vi "Dato_Booleano.vi"() -> ()   [LabVIEW 2016]
panel:
  in  "Boolean":bool
  in  "Stop Button":bool
  in  "STR1":string
  in  "DBL1":dbl
  in  "ARRAY1":dbl[](array[numeric])
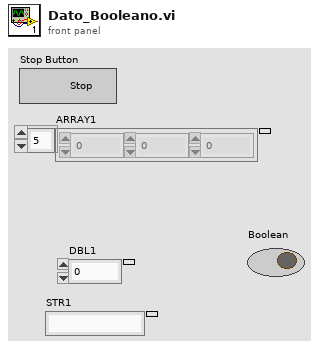
[diagram p1: front panel]
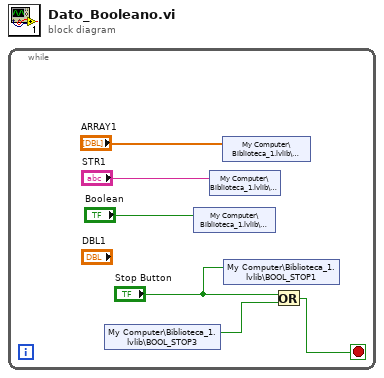
[diagram p0: block diagram]
diagram:
  n1 = while {
    stop <- w4 stop-if-true
    n2 = shared-variable "My Computer\\Biblioteca_1.lvlib\\BOOL_STOP3"() -> (w5:bool)  [unwired: 1 in, 1 out]
    n3 = shared-variable "My Computer\\Biblioteca_1.lvlib\\BOOL3"("Boolean") -> ()  [unwired: 1 in, 1 out]
    n4 = shared-variable "My Computer\\Biblioteca_1.lvlib\\STR1"("STR1") -> ()  [unwired: 1 in, 1 out]
    n5 = shared-variable "My Computer\\Biblioteca_1.lvlib\\ARRAY1"("ARRAY1") -> ()  [unwired: 1 in, 1 out]
    n6 = shared-variable "My Computer\\Biblioteca_1.lvlib\\BOOL_STOP1"("Stop Button") -> ()  [unwired: 1 in, 1 out]
    n7 = Or(x="Stop Button", y=w5) -> (x .or. y?=w4:bool)
  }
